vi "Read Alias.vi"(8 "error in":errorcluster, 11 "Plugin_Channels in":refnum<class "Plugin_Channels.lvclass">) -> (0 "error out":errorcluster, 2 "Alias":string, 3 "Plugin_Channels out":refnum<class "Plugin_Channels.lvclass">)   [LabVIEW 2020, in "Plugin.lvlib" / "Plugin_Channels.lvclass"]
doc: "Reads the alias name"
uses:
  Plugin_Channels.lvclass
panel:
  out "initialized array":string[](array[string])
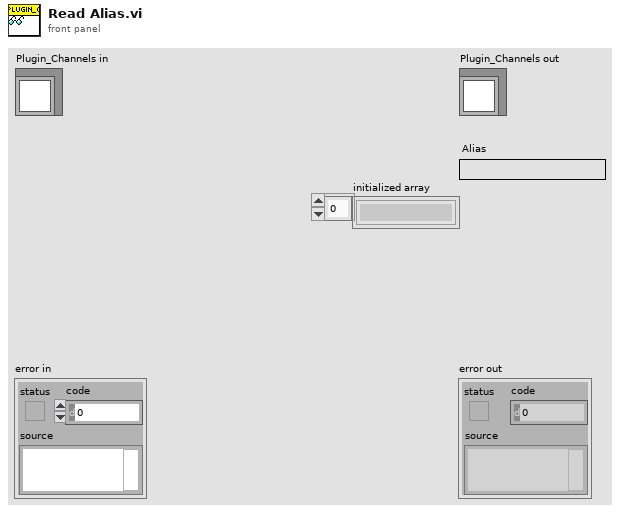
[diagram p1: front panel]
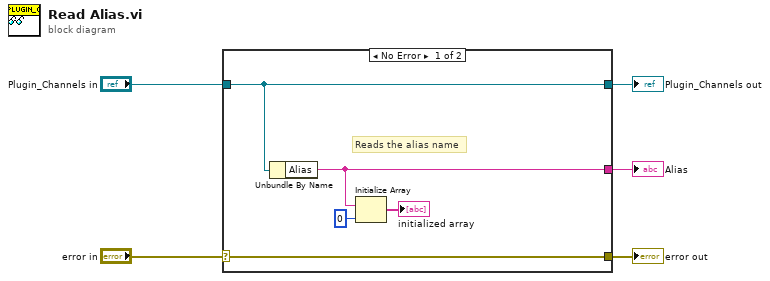
[diagram p0: block diagram]
diagram:
  n1 = case shown="No Error" "error in" {
    selector: "error in" -> [w10 w11]
    tunnel: [w10 w11] -> w4
    tunnel: [w9 w12] -> w2
    tunnel: "Plugin_Channels in" -> [w9 w12]
    tunnel: [w8 _] -> w1
    frame No Error {
      # "Reads the alias name"
      n2 = Unbundle By Name(w9) -> ("Alias"=w8:string)
      n3 = Initialize Array(w8, 0 ("dimension size")) -> (→"initialized array":string[])
    }
    frame Error {
    }
  }
  "error out" <- w4
  "Plugin_Channels out" <- w2
  "Alias" <- w1
